vi "searchNode.vi"(8 "error in (no error)":errorcluster, 9 "searchElementName":string, 10 "searchElementIn":string, 11 "xmlNode in":refnum<class "xmlNode.lvclass">) -> (0 "error out":errorcluster, 2 "arrayXmlNodes":refnum<class "xmlNode.lvclass">[][](array[class]), 3 "xmlNode out":refnum<class "xmlNode.lvclass">)   [LabVIEW 2009, in "Tools.lvlib" / "xml.lvlib" / "xmlNode.lvclass"]
doc: "Searchs for an xml node, gives back a 2D array."
uses:
  xmlNode.lvclass
  XmlParser.lvclass
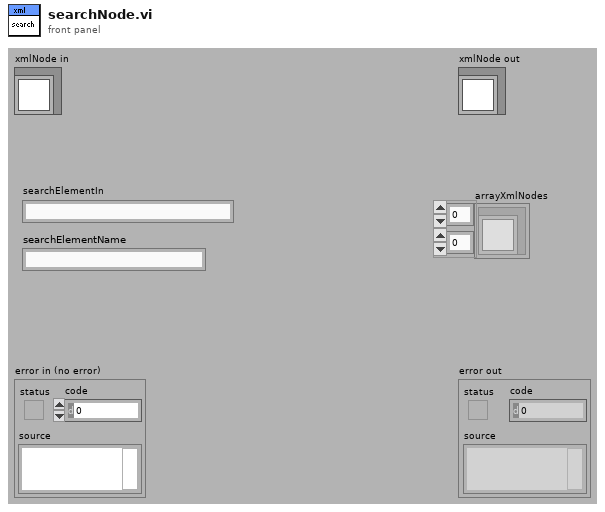
[diagram p1: front panel]
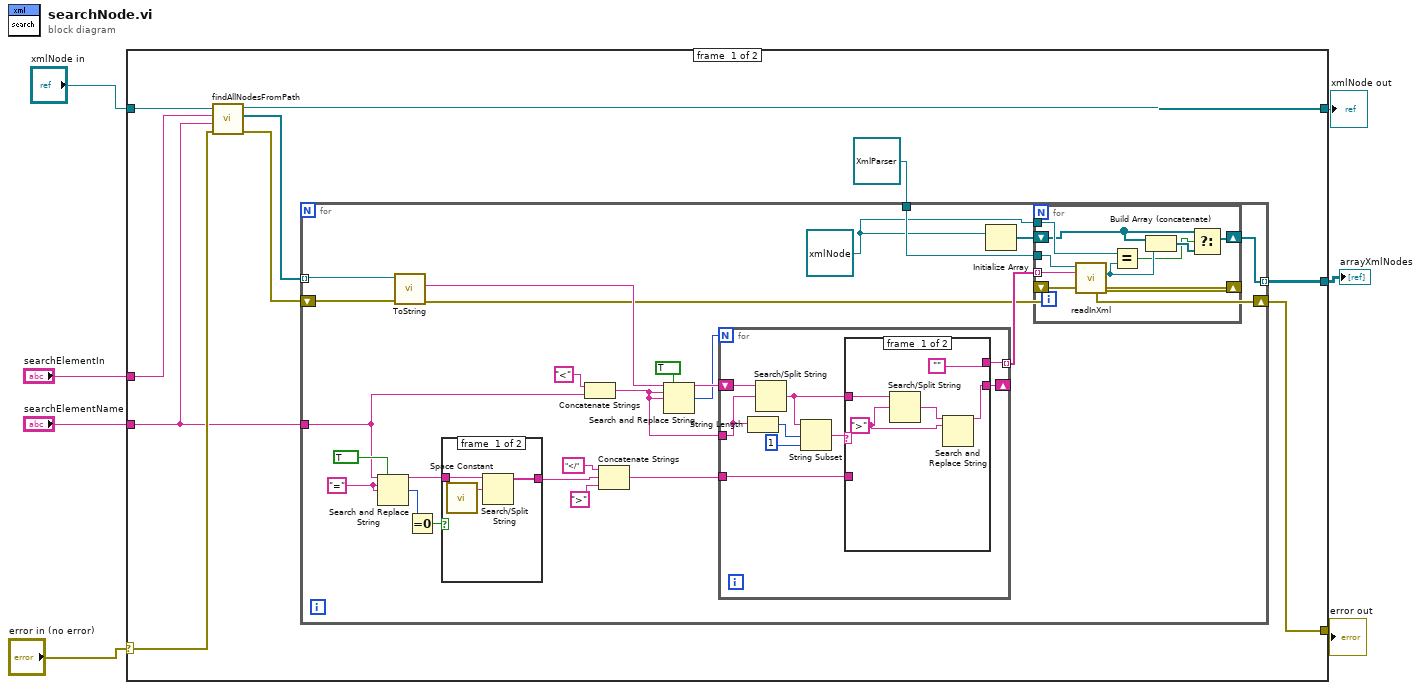
[diagram p0: block diagram]
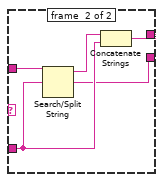
[diagram p2: hidden frame]
diagram:
  n1 = case shown="No Error" "error in (no error)" {
    selector: "error in (no error)" -> [w15 w77]
    tunnel: [w9 w77] -> w6
    tunnel: [w16 w76] -> w4
    tunnel: "xmlNode in" -> [w17 w76]
    tunnel: "searchElementIn" -> [w14 _]
    tunnel: "searchElementName" -> [w13 _]
    tunnel: [w8 _] -> w1
    frame #0 {
      n2 = call "findAllNodesFromPath.vi"("error in (no error)"=w15, "searchElement"=w13, "nodePath"=w14, "xmlNode in"=w17) -> ("error out"=w12:errorcluster, "arrayXmlNodes"=w10:refnum<class "xmlNode.lvclass">[], "xmlNode out"=w16:refnum<class "xmlNode.lvclass">)  [unwired: 5 in]
      n3 = for {
        tunnel: w13 -> [w28]
        tunnel: w10 -> [w27] mode=indexing
        tunnel: [w18] -> w8 mode=indexing
        shift-right: [w23] -> w9
        shift-left: w12 -> [w26]
        tunnel: refnum<class "XmlParser.lvclass"> refnum ("Tools.lvlib:XmlParser.lvclass") -> [w20]
        w19 = refnum<class "xmlNode.lvclass"> refnum ("Tools.lvlib:xml.lvlib:xmlNode.lvclass")
        w39 = "="
        n4 = Search and Replace String(replace all?=TRUE, input string=w28, search string=w39, replace string=w39) -> (result string=w36:string, number of replacements=w38:i32)  [unwired: 4 in, 2 out]
        n5 = call-dynamic "ToString.vi"("error in (no error)"=w26, "xmlNode in"=w27) -> ("error out"=w22:errorcluster, "xml"=w25:string)  [unwired: 7 in, 1 out]
        n6 = Equal To 0?(x=w38) -> (x = 0?=w37:bool)
        n7 = case shown="False" w37 {
          tunnel: w36 -> [w74 w75]
          tunnel: [w72 w75] -> w34
          frame #0 {
            n8 = call <vilib>:"Space Constant.vi"() -> ("String"=w73:string)
            n9 = Search/Split String(string=w74, search string/char (-)=w73) -> (substring before match=w72:string)  [unwired: 1 in, 2 out]
          }
          frame #1 {
          }
        }
        n10 = Concatenate Strings("<", w28) -> (w32:string)
        n11 = Concatenate Strings("</", w34, ">") -> (w31:string)
        n12 = Search and Replace String(replace all?=TRUE, input string=w25, search string=w32, replace string=w32) -> (result string=w30:string, number of replacements=w29:i32)  [unwired: 4 in, 2 out]
        n13 = for {
          N: w29 -> [_]
          tunnel: w32 -> [w53]
          tunnel: w31 -> [w60]
          shift-right: [w59] -> _
          shift-left: w30 -> [w61]
          tunnel: [w58] -> w24 mode=indexing
          n14 = String Length(string=w53) -> (length=w54:i32)
          n15 = Search/Split String(string=w61, search string/char (-)=w53) -> (match + rest of string=w55:string)  [unwired: 1 in, 2 out]
          n16 = String Subset(string=w55, offset (0)=w54, length (rest)=1) -> (substring=w57:string)
          n17 = case shown="\" \", \">\"" w57 {
            tunnel: w60 -> [_ w71]
            tunnel: [w63 w69] -> w59
            tunnel: ["" w68] -> w58
            tunnel: w55 -> [w66 w67]
            frame #0 {
              w64 = ">"
              n18 = Search/Split String(string=w66, search string/char (-)=w64) -> (match + rest of string=w65:string)  [unwired: 1 in, 2 out]
              n19 = Search and Replace String(input string=w65, search string=w64) -> (result string=w63:string)  [unwired: 6 in, 3 out]
            }
            frame #1 {
              n20 = Search/Split String(string=w67, search string/char (-)=w71) -> (substring before match=w70:string, match + rest of string=w69:string)  [unwired: 1 in, 1 out]
              n21 = Concatenate Strings(w70, w71) -> (w68:string)
            }
          }
        }
        n22 = Initialize Array(w19) -> (w21:refnum<class "xmlNode.lvclass">[])  [unwired: 1 in]
        n23 = for {
          tunnel: w20 -> [w52]
          tunnel: w24 -> [w49] mode=indexing
          shift-right: [w50] -> w23
          shift-left: w22 -> [w51]
          shift-right: [w43] -> w18
          shift-left: w21 -> [w47]
          tunnel: w19 -> [w48]
          n24 = call "readInXml.vi"("error in (no error)"=w51, "xmlString"=w49, "XmlParser in"=w52) -> ("error out"=w50:errorcluster, "xmlNode"=w46:refnum<class "xmlNode.lvclass">)  [unwired: 6 in, 1 out]
          n25 = Equal?(x=w48, y=w46) -> (x = y?=w44:bool)
          n26 = Build Array (concatenate)(w47, w46) -> (w45:refnum<class "xmlNode.lvclass">[])
          n27 = Select(t=w47, s=w44, f=w45) -> (s? t:f=w43:refnum<class "xmlNode.lvclass">[])
        }
      }
    }
    frame #1 {
    }
  }
  "error out" <- w6
  "xmlNode out" <- w4
  "arrayXmlNodes" <- w1
